vi "RegSolver.vi"(6 "Display Precision":i32=3 min=0, 7 "Models":T2(radio), 8 "Fitting method":u16(ring) items=["Least Square", "Least Absolute Residual", "Bisquare"], 9 "Order":i32=2, 10 "Y Data":dbl[](array[numeric]), 11 "X Data":dbl[](array[numeric])) -> (0 "error information":string, 1 "Equation of fit":string, 2 "Fitted Data":dbl[](array[numeric]) format="%#.6g", 3 "XY Graph":T1(graph), 4 "MSE":dbl format="%#.3g")   [LabVIEW 2014]
doc: "Demonstrates how to use the linear, polynomial, exponential, and power Fitting VIs for selected data sets."
uses:
  <vilib>/Analysis/NI_AALPro.lvlib
  <vilib>/Utility/error.llb/DialogType.ctl
  <vilib>/gmath/NI_Gmath.lvlib
panel:
  # "I only changed the example vi, Regression Solver.vi, into a sub vi. Thank you NI or LabView for your examples!\n\nOverview: Demonstrates fitting data to linear, polynomial, exponential and power models with the Fitting VIs.\nRequirements: LabVIEW Full Development System\nInstructions: \n1. Run the VI. \n2. Select different Models and notice the changes to the graph and MSE.\n3. Click Stop to stop the VI."
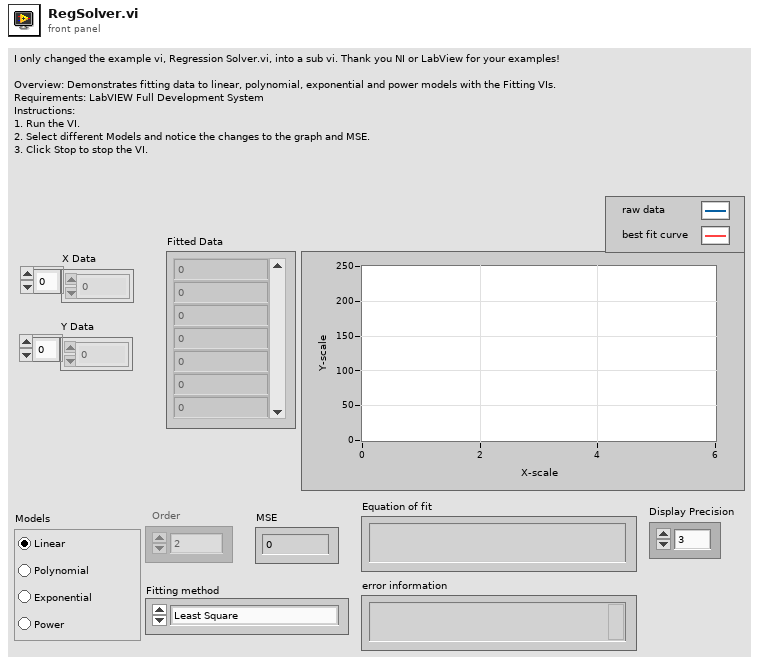
[diagram p1: front panel]
types:
  T1 = cluster{"Data":dbl[], "Best Exponential Fit":dbl[]}[]
  T2 = enum32{"Linear", "Polynomial", "Exponential", "Power"}
  T3 = enum8{"Enabled", "Disabled", "Disabled and Grayed Out"}
  T4 = typedef "DialogType.ctl" = u16
  T5 = enum16{"Linear", "Polynomial", "Exponential", "Power"}
  T6 = cluster{"amp min":dbl, "amp max":dbl, "damping min":dbl, "damping max":dbl, "offset min":dbl, "offset max":dbl}
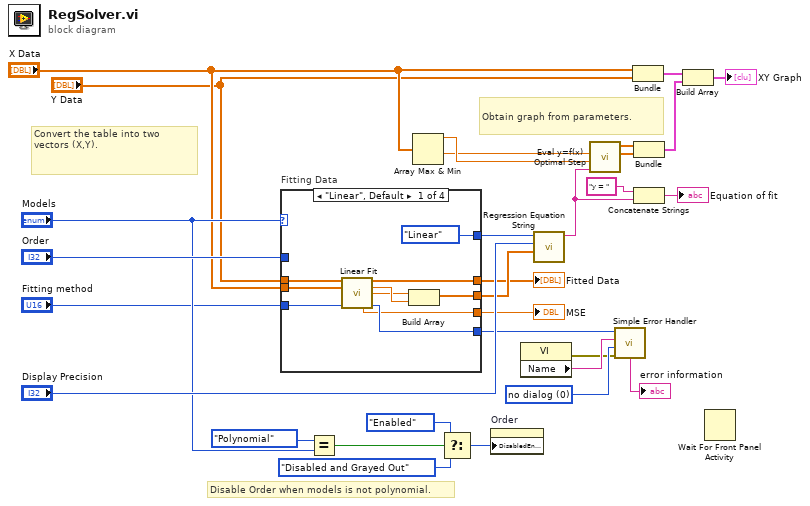
[diagram p0: block diagram]
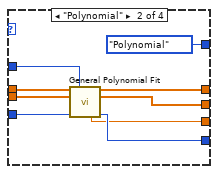
[diagram p2: hidden frame]
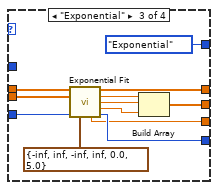
[diagram p3: hidden frame]
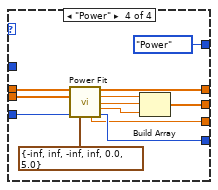
[diagram p4: hidden frame]
diagram:
  w24 = T4 0 items=["no dialog", "OK message", "continue or stop message", "OK message + warnings", "continue/stop + warnings"] ("type of dialog (OK msg:1)")
  # "Convert the table into two vectors (X,Y)."
  # "Disable Order when models is not polynomial."
  # "Obtain graph from parameters."
  n1 = case "Fitting Data" shown="\"Linear\", Default" "Models" {
    tunnel: [w40 w49 w59 w72] -> w28
    tunnel: "Y Data" -> [w39 w48 w60 w64]
    tunnel: "X Data" -> [w37 w47 w61 w73]
    tunnel: [w33 w46 w58 w71] -> w27
    tunnel: [w38 w45 w57 w70] -> w22
    tunnel: [w34 w44 w54 w67] -> w23
    tunnel: "Order" -> [_ w43 _ _]
    tunnel: "Fitting method" -> [w32 w42 w51 w65]
    tunnel: [T5."Linear" ("fit type") T5."Polynomial" ("fit type") T5."Exponential" ("fit type") T5."Power" ("fit type")] -> w6
    frame "Linear", Default {
      n2 = call <vilib>:"Linear Fit.vi"("Y"=w39, "X"=w37, "method"=w32) -> ("Best Linear Fit"=w38:dbl[], "slope"=w36:dbl, "intercept"=w35:dbl, "residue"=w33:dbl, "error"=w40:i32)  [unwired: 8 in]
      n3 = Build Array(w35, w36) -> (w34:dbl[])
    }
    frame "Polynomial" {
      n4 = call <vilib>:"General Polynomial Fit.vi"("Y"=w48, "polynomial order"=w43, "X"=w47, "method"=w42) -> ("Best Polynomial Fit"=w45:dbl[], "Polynomial Coefficients"=w44:dbl[], "residue"=w46:dbl, "error"=w49:i32)  [unwired: 8 in]
    }
    frame "Exponential" {
      n5 = call <vilib>:"Exponential Fit.vi"("Y"=w60, "X"=w61, "method"=w51, "parameter bounds"=T6 {"amp min"=-inf, "amp max"=inf, "damping min"=-inf, "damping max"=inf, "offset min"=0.0, "offset max"=5.0}) -> ("Best Exponential Fit"=w57:dbl[], "amplitude"=w55:dbl, "damping"=w56:dbl, "offset"=w53:dbl, "residue"=w58:dbl, "error"=w59:i32)  [unwired: 6 in]
      n6 = Build Array(w55, w56, w53) -> (w54:dbl[])
    }
    frame "Power" {
      n7 = call <vilib>:"Power Fit.vi"("Y"=w64, "X"=w73, "method"=w65, "parameter bounds"=T6 {"amp min"=-inf, "amp max"=inf, "damping min"=-inf, "damping max"=inf, "offset min"=0.0, "offset max"=5.0}) -> ("Best Power Fit"=w70:dbl[], "amplitude"=w68:dbl, "power"=w69:dbl, "offset"=w66:dbl, "residue"=w71:dbl, "error"=w72:i32)  [unwired: 6 in]
      n8 = Build Array(w68, w69, w66) -> (w67:dbl[])
    }
  }
  "Fitted Data" <- w22
  "MSE" <- w27
  n9 = Equal?(x=T2."Polynomial", y="Models") -> (x = y?=w19:bool)
  n10 = Array Max & Min(array="X Data") -> (max value=w11:dbl, min value=w7:dbl)  [unwired: 2 out]
  n11 = Select(t=T3."Enabled" ("Disabled"), s=w19, f=T3."Disabled and Grayed Out" ("Disabled")) -> (s? t:f=w16:T3)
  n12 = property on="Order" class="DigNum (strict)"("DisabledEnum"=w16) -> ()  [unwired: 2 in, 2 out]
  n13 = property class="VI"() -> (error out=w3:errorcluster, "Name"=w4:string)  [unwired: 2 in, 1 out]
  n14 = call "Regression Equation String.vi"("coefficients"=w23, "precision"="Display Precision", "fit type"=w6) -> ("Formula"=w8:string)  [unwired: 8 in]
  n15 = call <vilib>:"Eval y=f(x) Optimal Step.vi"("formula"=w8, "end"=w11, "start"=w7) -> ("Y Values"=w14:dbl[], "X Values"=w15:dbl[])  [unwired: 2 in, 2 out]
  n16 = call <vilib>:"Simple Error Handler.vi"("error code (no error:0)"=w28, "error source (\" \")"=w4, "type of dialog (OK msg:1)"=w24, "error in (no error)"=w3) -> ("message"=→"error information":string)  [unwired: 1 in, 4 out]
  n17 = Bundle("X Data"="X Data", "Y Data"="Y Data") -> (w25:cluster{"X Data":dbl[], "Y Data":dbl[]})  [unwired: 1 in]
  n18 = Bundle("X Values"=w15, "Y Values"=w14) -> (w21:cluster{"X Values":dbl[], "Y Values":dbl[]})  [unwired: 1 in]
  n19 = Concatenate Strings("y = " ("string"), w8) -> (→"Equation of fit":string)
  n20 = Build Array(w25, w21) -> (→"XY Graph":cluster{"X Values":dbl[], "Y Values":dbl[]}[])
  n21 = Wait For Front Panel Activity() -> ()  [unwired: 3 in, 1 out]
